vi "Scripting_LvClassConstantToClassType.vi"(11 "Value":variant) -> (0 "ClassPath":path, 1 "FullQualifiedClassName'sDataMember":string, 2 "JustClassName":string, 3 "FullQualifiedClassName":string)   [LabVIEW 2014]
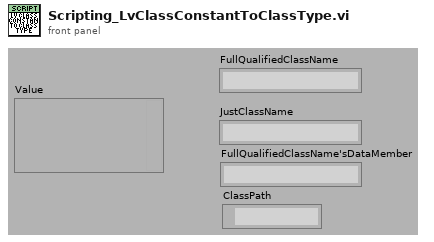
[diagram p1: front panel]
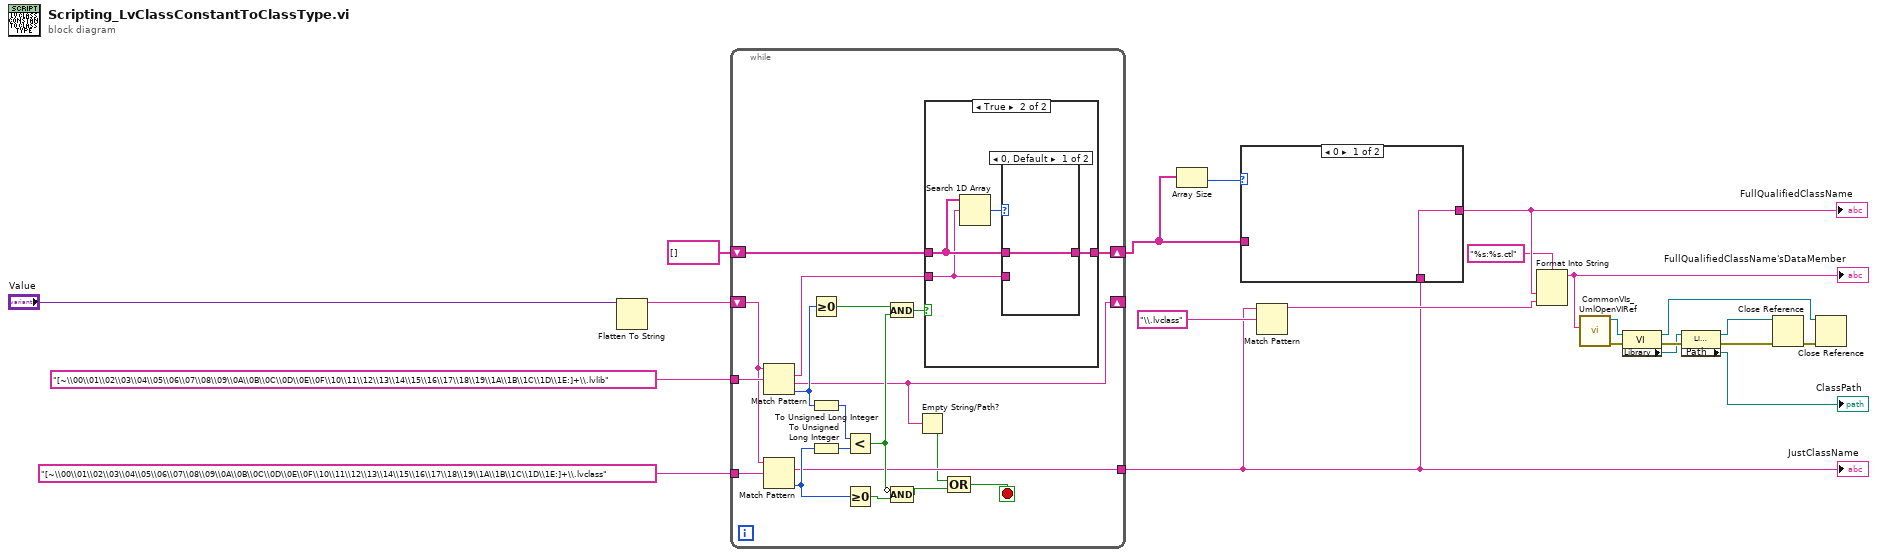
[diagram p0: block diagram]
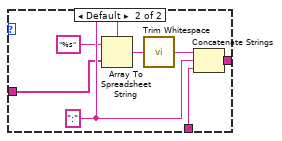
[diagram p2: hidden frame]
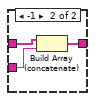
[diagram p4: hidden frame]
diagram:
  n1 = Flatten To String(anything="Value") -> (data string=w21:string)  [unwired: 3 in, 2 out]
  n2 = while {
    shift-right: [w24] -> _
    shift-left: w21 -> [w40]
    tunnel: "[~\\00\\01\\02\\03\\04\\05\\06\\07\\08\\09\\0A\\0B\\0C\\0D\\0E\\0F\\10\\11\\12\\13\\14\\15\\16\\17\\18\\19\\1A\\1B\\1C\\1D\\1E:]+\\.lvlib" ("regular expression 2") -> [w41]
    tunnel: "[~\\00\\01\\02\\03\\04\\05\\06\\07\\08\\09\\0A\\0B\\0C\\0D\\0E\\0F\\10\\11\\12\\13\\14\\15\\16\\17\\18\\19\\1A\\1B\\1C\\1D\\1E:]+\\.lvclass" ("regular expression") -> [w39]
    shift-right: [w31] -> w2
    shift-left: string[] [] -> [w32]
    tunnel: [w27] -> w13
    stop <- w25 stop-if-true
    n3 = Match Pattern(string=w40, regular expression=w41) -> (match substring=w30:string, after substring=w24:string, offset past match=w36:i32)  [unwired: 1 in, 1 out]
    n4 = Match Pattern(string=w40, regular expression=w39) -> (match substring=w27:string, offset past match=w35:i32)  [unwired: 1 in, 2 out]
    n5 = Greater Or Equal To 0?(x=w36) -> (x >= 0?=w34:bool)
    n6 = To Unsigned Long Integer(number=w36) -> (unsigned 32bit integer=w38:u32)
    n7 = To Unsigned Long Integer(number=w35) -> (unsigned 32bit integer=w37:u32)
    n8 = Less?(x=w38, y=w37) -> (x < y?=w29:bool)
    n9 = Greater Or Equal To 0?(x=w35) -> (x >= 0?=w28:bool)
    n10 = And(x=w34, y=w29) -> (x .and. y?=w33:bool)
    n11 = Compound Arithmetic op=AND(invert w29, w28) -> (w26:bool)
    n12 = Empty String/Path?(string/path=w24) -> (empty?=w23:bool)
    n13 = case shown="True" w33 {
      tunnel: w32 -> [w42 w45]
      tunnel: [w42 w46] -> w31
      tunnel: w30 -> [_ w44]
      frame False {
      }
      frame True {
        n14 = Search 1D Array(1D array=w45, element=w44) -> (index of element=w43:i32)  [unwired: 1 in]
        n15 = case shown="0, Default" w43 {
          tunnel: [w47 w50] -> w46
          tunnel: w45 -> [w47 w49]
          tunnel: w44 -> [_ w48]
          frame 0, Default {
          }
          frame -1 {
            n16 = Build Array (concatenate)(w49, w48) -> (w50:string[])
          }
        }
      }
    }
    n17 = Compound Arithmetic op=OR(w23, w26) -> (w25:bool)
  }
  "JustClassName" <- w13
  n18 = Array Size(array=w2) -> (size(s)=w1:i32)
  n19 = case shown="0" w1 {
    tunnel: [w51 w58] -> w22
    tunnel: w13 -> [w51 w53]
    tunnel: w2 -> [_ w52]
    frame 0 {
    }
    frame Default {
      w57 = ":" ("delimiter (Tab)")
      n20 = Array To Spreadsheet String(delimiter (Tab)=w57, array=w52, 3:"%s" ("format string")) -> (spreadsheet string=w55:string)
      n21 = call <vilib>:"Trim Whitespace.vi"("string"=w55) -> ("trimmed string"=w56:string)  [unwired: 1 in]
      n22 = Concatenate Strings(w56, w57, w53) -> (w58:string)
    }
  }
  "FullQualifiedClassName" <- w22
  n23 = Match Pattern(string=w13, regular expression="\\.lvclass") -> (before substring=w17:string)  [unwired: 1 in, 3 out]
  n24 = Format Into String(format string="%s:%s.ctl", w22, w17) -> (resulting string=w3:string)  [unwired: 2 in, 1 out]
  "FullQualifiedClassName'sDataMember" <- w3
  n25 = call <resource>:"CommonVIs_UmlOpenVIRef.vi"("ViPath/ViName"=w3) -> ("error out"=w4:errorcluster, "vi reference"=w5:refnum<vi>)  [unwired: 7 in, 2 out]
  n26 = property class="VI"(reference=w5, error in=w4) -> (reference out=w6:refnum<vi>, error out=w11:errorcluster, "Library"=w10:refnum<vi>)
  n27 = property class="Library"(reference=w10, error in=w11) -> (reference out=w8:refnum<vi>, error out=w9:errorcluster, "Path"=→"ClassPath":path)
  n28 = Close Reference(reference=w8, error in (no error)=w9) -> (error out=w7:errorcluster)
  n29 = Close Reference(reference=w6, error in (no error)=w7) -> ()  [unwired: 1 out]
